vi "CompressorControlLoop.vi"(8 "error in (no error)":errorcluster, 11 "CompressorDevRef":T1={"DevStatus"={"status"=FALSE, "code"=0, "source"=""}, "DigitalInputDevRef"={"DevStatus"={"status"=FALSE, "code"=0, "source"=""}, "DIO Channel"=enum."Invalid", "Digital Module"=enum."Digital Module 1"}, "RelayDevRef"={"DevStatus"={"status"=FALSE, "code"=0, "source"=""}, "Relay Channel"=enum."Invalid", "Digital Module"=enum."Digital Module 1", "Relay Direction"=enum."Both directions"}}) -> ()   [LabVIEW 2013]
doc: "Monitors the pressure switch and updates the relay of up to two compressors. Use the Start, Stop, and GetEnableState VIs to update the compressor state. Use this VI in parallel with the rest of the robot code. Do not place this VI in another loop or in the Teleop code.\n\nThis software is licensed. Open the labview\\readme\\WPI Robotics Library Open Source License.txt file for more information."
uses:
  <vilib>/Rock Robotics/WPI/Compressor/WPI_CompressorDevRef.ctl
  <vilib>/Rock Robotics/WPI/DigitalInput/WPI_DigitalInputDevRef.ctl
  <vilib>/Rock Robotics/SystemInterfaces/DIO/FPGA_DIOChannel.ctl
  <vilib>/Rock Robotics/SystemInterfaces/Typedef/FPGA_TypedefDigitalModule.ctl
  <vilib>/Rock Robotics/WPI/Relay/WPI_RelayDevRef.ctl
  <vilib>/Rock Robotics/SystemInterfaces/DIO/FPGA_DIORelayChannel.ctl
  <vilib>/Rock Robotics/WPI/Relay/WPI_RelayDirection.ctl
  <vilib>/Rock Robotics/WPI/Relay/WPI_RelayValue.ctl
panel:
  # "This VI loops and doesn't return.\nPlacing it into another loop will\nprevent that loop from iterating.\n\nPeriodic tasks is a good location for it."
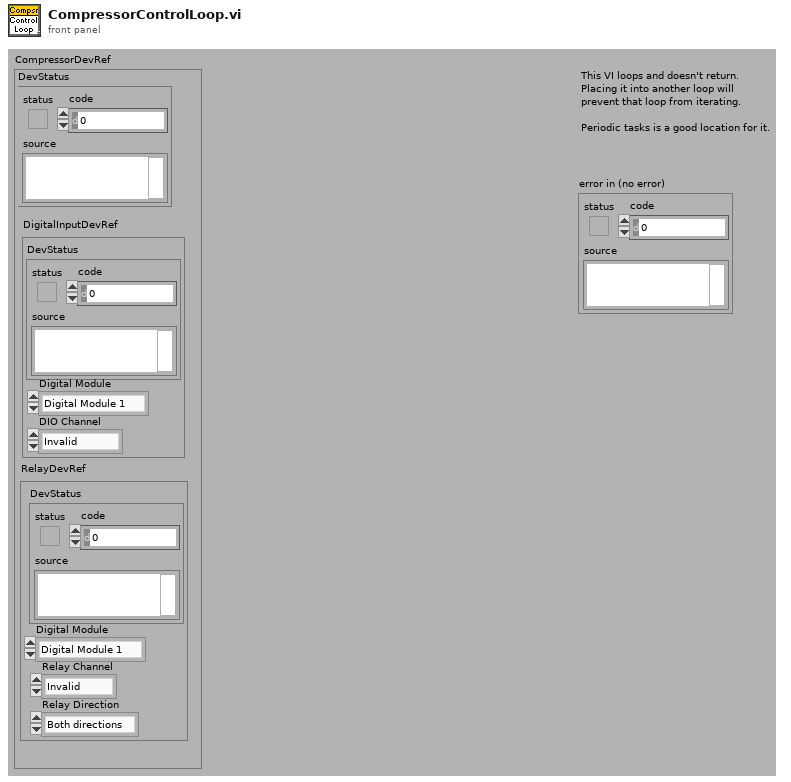
[diagram p1: front panel]
types:
  T1 = typedef "WPI_CompressorDevRef.ctl" = cluster{"DevStatus":errorcluster, "DigitalInputDevRef":T2, "RelayDevRef":T5}
  T2 = typedef "WPI_DigitalInputDevRef.ctl" = cluster{"DevStatus":errorcluster, "DIO Channel":T3, "Digital Module":T4}
  T3 = typedef "FPGA_DIOChannel.ctl" = enum8{"DIO 1", "DIO 2", "DIO 3", "DIO 4", "DIO 5", "DIO 6", "DIO 7", "DIO 8", "DIO 9", "DIO 10", "DIO 11", "DIO 12", "DIO 13", "DIO 14", "Invalid"}
  T4 = typedef "FPGA_TypedefDigitalModule.ctl" = enum16{"Digital Module 1", "Digital Module 2"}
  T5 = typedef "WPI_RelayDevRef.ctl" = cluster{"DevStatus":errorcluster, "Relay Channel":T6, "Digital Module":T4, "Relay Direction":T7}
  T6 = typedef "FPGA_DIORelayChannel.ctl" = enum8{"Relay 1", "Relay 2", "Relay 3", "Relay 4", "Relay 5", "Relay 6", "Relay 7", "Relay 8", "Invalid"}
  T7 = typedef "WPI_RelayDirection.ctl" = enum16{"Both directions", "Forward only", "Reverse only"}
  T8 = typedef "WPI_RelayValue.ctl" = enum16{"Off", "On", "Forward", "Reverse"}
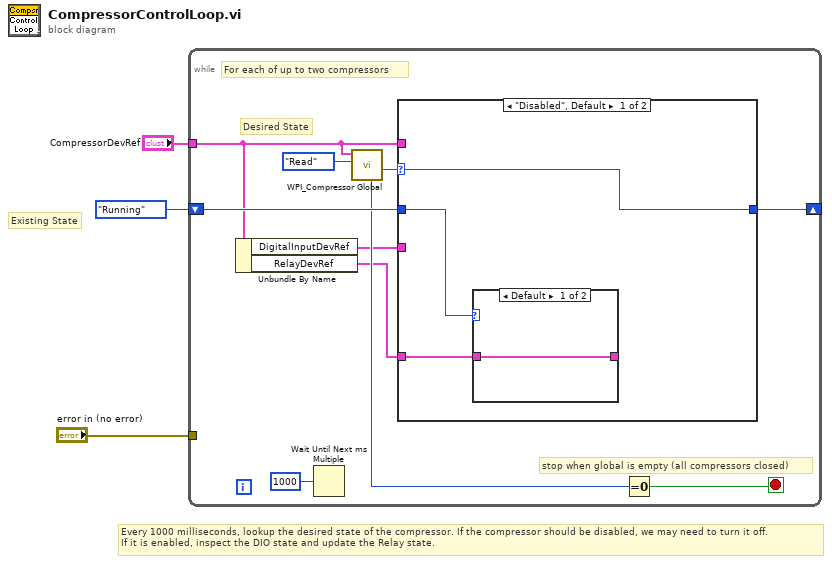
[diagram p0: block diagram]
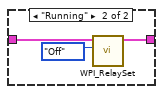
[diagram p2: hidden frame]
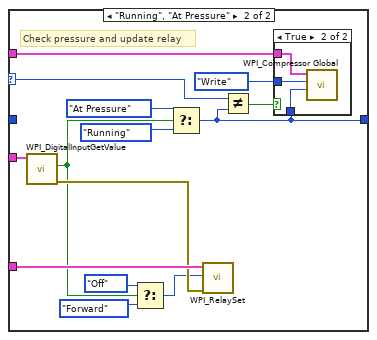
[diagram p3: hidden frame]
diagram:
  # "Every 1000 milliseconds, lookup the desired state of the compressor. If the compressor should be disabled, we may need to turn it off.\nIf it is enabled, inspect the DIO state and update the Relay state."
  # "Existing State"
  n1 = while {
    shift-right: [w11] -> _
    shift-left: enum16{"Disabled", "Running", "At Pressure"}."Running" ("Compressor State") -> [w12]
    tunnel: "error in (no error)" -> [_]
    tunnel: "CompressorDevRef" -> [w10]
    stop <- w8 stop-if-true
    # "Desired State"
    # "stop when global is empty (all compressors closed)"
    # "For each of up to two compressors"
    n2 = Unbundle By Name(w10) -> ("DigitalInputDevRef"=w5:T2, "RelayDevRef"=w4:T5)
    n3 = Wait Until Next ms Multiple(millisecond multiple=u32 1000 ("timeout in ms (0)")) -> ()  [unwired: 1 out]
    n4 = call <vilib>:"WPI_Compressor Global.vi"("Operation"=enum16{"Read", "Write", "Add", "Remove"}."Read", "CompressorDevRef"=w10) -> ("Compressor State Out"=w6:enum16{"Disabled", "Running", "At Pressure"}, "Compressor Count"=w9:u8)  [unwired: 8 in]
    n5 = case shown="\"Disabled\", Default" w6 {
      selector: w6 -> [w14 w21]
      tunnel: w5 -> [_ w34]
      tunnel: w4 -> [w16 w33]
      tunnel: w12 -> [w15 _]
      tunnel: [w14 w22] -> w11
      tunnel: w10 -> [_ w24]
      frame "Disabled", Default {
        n6 = case shown="Default" w15 {
          tunnel: w16 -> [w17 w19]
          tunnel: [w17 w18] -> _
          frame Default {
          }
          frame "Running" {
            n7 = call <vilib>:"WPI_RelaySet.vi"("RelayValue"=WPI_RelayValue."Off", "RelayDevRef"=w19) -> ("RelayDevRef"=w18:T5)  [unwired: 1 in, 8 out]
          }
        }
      }
      frame "Running", "At Pressure" {
        # "Check pressure and update relay"
        n8 = call <vilib>:"WPI_DigitalInputGetValue.vi"("DigitalInputDevRef"=w34) -> ("error out"=w32:errorcluster, "Value"=w28:bool)  [unwired: 1 in, 8 out]
        n9 = Select(t=WPI_RelayValue."Off" ("RelayValue"), s=w28, f=WPI_RelayValue."Forward" ("RelayValue")) -> (s? t:f=w29:T8)
        n10 = Select(t=enum16{"Disabled", "Running", "At Pressure"}."At Pressure" ("Compressor State"), s=w28, f=enum16{"Disabled", "Running", "At Pressure"}."Running" ("Compressor State")) -> (s? t:f=w22:enum16{"Disabled", "Running", "At Pressure"})
        n11 = call <vilib>:"WPI_RelaySet.vi"("error in (no error)"=w32, "RelayValue"=w29, "RelayDevRef"=w33) -> ()  [unwired: 9 out]
        n12 = Not Equal?(x=w21, y=w22) -> (x != y?=w23:bool)
        n13 = case shown="True" w23 {
          tunnel: w22 -> [_ w37]
          tunnel: enum16{"Read", "Write", "Add", "Remove"}."Write" ("Operation") -> [_ w36]
          tunnel: w24 -> [_ w35]
          frame False {
          }
          frame True {
            n14 = call <vilib>:"WPI_Compressor Global.vi"("Compressor State In"=w37, "Operation"=w36, "CompressorDevRef"=w35) -> ()  [unwired: 7 in, 2 out]
          }
        }
      }
    }
    n15 = Equal To 0?(x=w9) -> (x = 0?=w8:bool)
  }
